vi "GetParameters.vi"(0 "Camera Reference in":refnum<k24>, 1 "error in (no error)":errorcluster) -> (2 "2D ExposureMode (Timed Auto HDR Flash)":enum16{"Timed", "Auto", "HDR", "Flash"}(ring), 3 "2D ExposureTime (0.1-999)":dbl=0.1 min=0.1 max=999.0 step=0.1, 4 "2D Gray Value":i32 min=1 max=999 step=1, 5 "2D Auto-Exposure ROI (x, y, width, height)":T2, 6 "2D Tone Mapping":bool, 7 "2D HDR Exposure Count":i32, 8 "2D HDR Exposure Sequence":T1, 9 "3D Exposure Multiplier":i32, 10 "3D Exposure Sequence":T3, 11 "3D Gain (0-16)":dbl, 12 "Depth Range (lower upper)":cluster{"lower":i32, "upper":i32}, 13 "ROI (x, y, width, height)":T2, 14 "Camera Reference out":refnum<k24>, 15 "error out":errorcluster, 16 "PointCloudSurfaceSmoothing (Off Weak Normal Strong)":u8(ring) items=["Off", "Weak", "Normal", "Strong"], 17 "PointCloudNoiseRemoval (Off Weak Normal Strong)":u8(ring) items=["Off", "Weak", "Normal", "Strong"], 18 "PointCloudOutlierRemoval (Off Weak Normal Strong)":u8(ring) items=["Off", "Weak", "Normal", "Strong"], 19 "Stripe Contrast Threshold (0-100)":i32 min=0 max=100 step=1)   [LabVIEW 2023]
uses:
  C:/Users/mech-mind/Downloads/LabView/MechEyeApiNet.dll
  MechEyeApiNet.dll
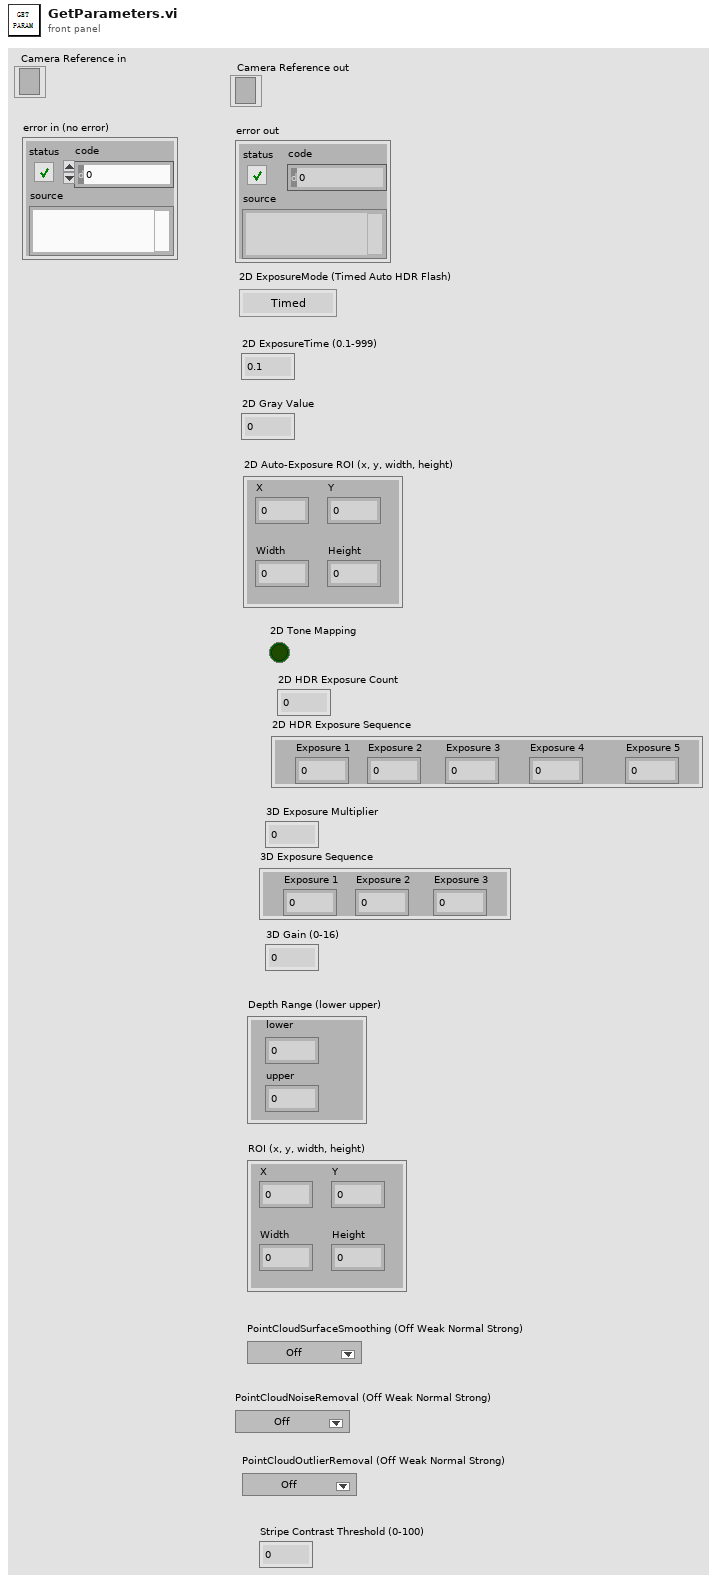
[diagram p1: front panel]
types:
  T1 = cluster{"Exposure 1":dbl, "Exposure 2":dbl, "Exposure 3":dbl, "Exposure 4":dbl, "Exposure 5":dbl}
  T2 = cluster{"X":i32, "Y":i32, "Width":i32, "Height":i32}
  T3 = cluster{"Exposure 1":dbl, "Exposure 2":dbl, "Exposure 3":dbl}
  T4 = cluster{"UpperLeftX":u32, "UpperLeftY":u32, "Width":u64, "Height":u64}
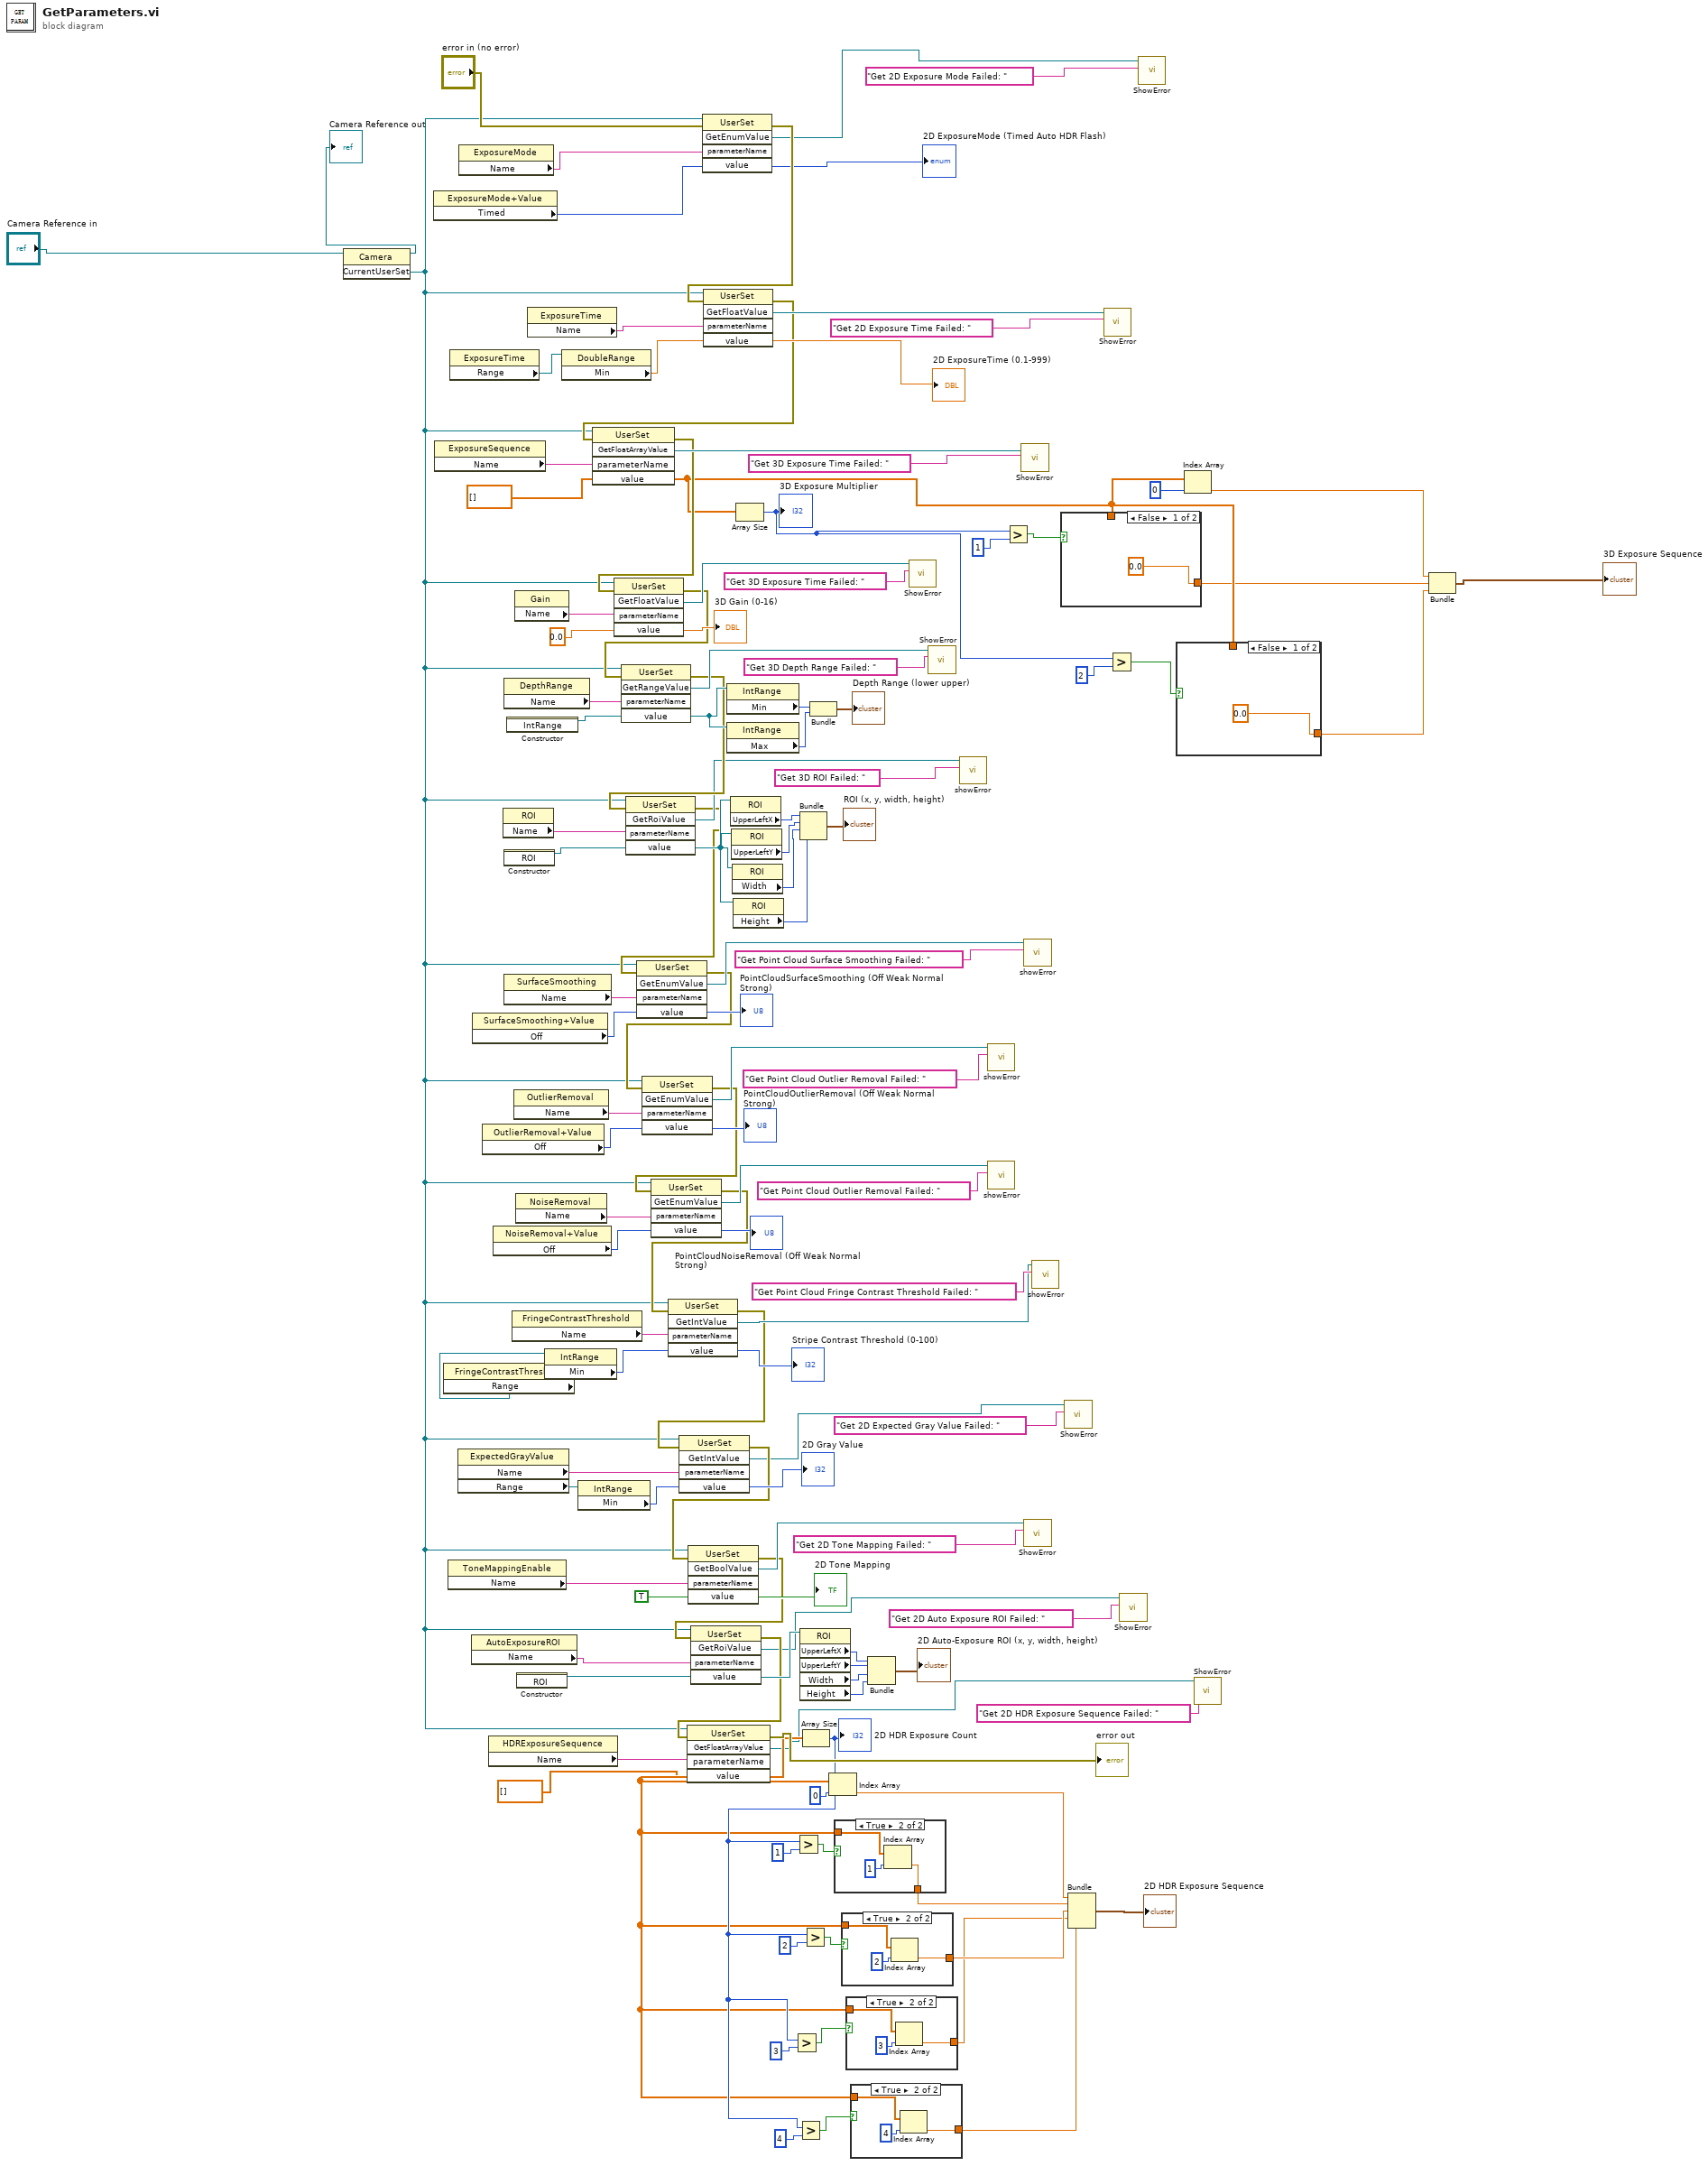
[diagram p0: block diagram]
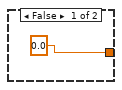
[diagram p2: hidden frame]
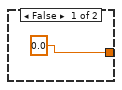
[diagram p3: hidden frame]
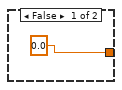
[diagram p4: hidden frame]
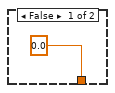
[diagram p5: hidden frame]
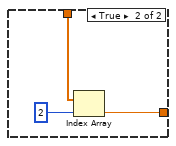
[diagram p6: hidden frame]
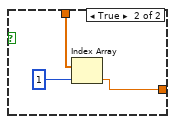
[diagram p7: hidden frame]
diagram:
  n1 = invoke class="Camera" method="CurrentUserSet"(reference="Camera Reference in") -> (reference out=→"Camera Reference out":refnum<k24>, "CurrentUserSet"=w25:refnum<k24>)  [unwired: 2 in, 1 out]
  n2 = property class="ExposureMode+Value"() -> ("Timed"=w120:i32)  [unwired: 2 in, 2 out]
  n3 = property class="ExposureSequence"() -> ("Name"=w117:string)  [unwired: 2 in, 2 out]
  n4 = property class="FringeContrastThreshold"() -> ("Range"=w63:refnum<k24>)  [unwired: 2 in, 2 out]
  n5 = property class="ToneMappingEnable"() -> ("Name"=w42:string)  [unwired: 2 in, 2 out]
  n6 = property class="ExposureTime"() -> ("Range"=w119:refnum<k24>)  [unwired: 2 in, 2 out]
  n7 = property class="ExpectedGrayValue"() -> ("Name"=w46:string, "Range"=w45:refnum<k24>)  [unwired: 2 in, 2 out]
  n8 = property class="ExposureMode"() -> ("Name"=w124:string)  [unwired: 2 in, 2 out]
  n9 = property class="AutoExposureROI"() -> ("Name"=w34:string)  [unwired: 2 in, 2 out]
  n10 = property class="SurfaceSmoothing+Value"() -> ("Off"=w86:i32)  [unwired: 2 in, 2 out]
  n11 = property class="OutlierRemoval+Value"() -> ("Off"=w80:i32)  [unwired: 2 in, 2 out]
  n12 = property class="HDRExposureSequence"() -> ("Name"=w24:string)  [unwired: 2 in, 2 out]
  n13 = property class="NoiseRemoval+Value"() -> ("Off"=w75:i32)  [unwired: 2 in, 2 out]
  n14 = property class="ROI"() -> ("Name"=w97:string)  [unwired: 2 in, 2 out]
  n15 = property class="DepthRange"() -> ("Name"=w108:string)  [unwired: 2 in, 2 out]
  n16 = constructor class="ROI"() -> (reference out=w96:refnum<k24>)  [unwired: 3 in, 2 out]
  n17 = property class="SurfaceSmoothing"() -> ("Name"=w87:string)  [unwired: 2 in, 2 out]
  n18 = constructor class="IntRange"() -> (reference out=w107:refnum<k24>)  [unwired: 3 in, 2 out]
  n19 = property class="FringeContrastThreshold"() -> ("Name"=w64:string)  [unwired: 2 in, 2 out]
  n20 = property class="OutlierRemoval"() -> ("Name"=w81:string)  [unwired: 2 in, 2 out]
  n21 = property class="Gain"() -> ("Name"=w111:string)  [unwired: 2 in, 2 out]
  n22 = property class="NoiseRemoval"() -> ("Name"=w76:string)  [unwired: 2 in, 2 out]
  n23 = constructor class="ROI"() -> (reference out=w27:refnum<k24>)  [unwired: 3 in, 2 out]
  n24 = property class="ExposureTime"() -> ("Name"=w122:string)  [unwired: 2 in, 2 out]
  n25 = property class="IntRange"(reference=w63) -> ("Min"=w62:i32)  [unwired: 1 in, 2 out]
  n26 = property class="DoubleRange"(reference=w119) -> ("Min"=w118:dbl)  [unwired: 1 in, 2 out]
  n27 = property class="IntRange"(reference=w45) -> ("Min"=w44:i32)  [unwired: 1 in, 2 out]
  n28 = invoke class="UserSet" method="GetEnumValue"(reference=w25, error in="error in (no error)", "parameterName"=w124, "value"=w120) -> (error out=w129:errorcluster, "GetEnumValue"=w126:refnum<k24>, "value"=→"2D ExposureMode (Timed Auto HDR Flash)":i32)  [unwired: 1 in, 2 out]
  n29 = invoke class="UserSet" method="GetFloatValue"(reference=w25, error in=w129, "parameterName"=w122, "value"=w118) -> (error out=w100:errorcluster, "GetFloatValue"=w125:refnum<k24>, "value"=→"2D ExposureTime (0.1-999)":dbl)  [unwired: 1 in, 2 out]
  n30 = invoke class="UserSet" method="GetFloatArrayValue"(reference=w25, error in=w100, "parameterName"=w117, "value"=dbl[] [] ("Array")) -> (error out=w99:errorcluster, "GetFloatArrayValue"=w114:refnum<k24>, "value"=w55:dbl[])  [unwired: 1 in, 2 out]
  n31 = invoke class="UserSet" method="GetFloatValue"(reference=w25, error in=w99, "parameterName"=w111, "value"=0.0) -> (error out=w98:errorcluster, "GetFloatValue"=w109:refnum<k24>, "value"=→"3D Gain (0-16)":dbl)  [unwired: 1 in, 2 out]
  n32 = invoke class="UserSet" method="GetRangeValue"(reference=w25, error in=w98, "parameterName"=w108, "value"=w107) -> (error out=w95:errorcluster, "GetRangeValue"=w101:refnum<k24>, "value"=w106:refnum<k24>)  [unwired: 1 in, 2 out]
  n33 = invoke class="UserSet" method="GetRoiValue"(reference=w25, error in=w95, "parameterName"=w97, "value"=w96) -> (error out=w71:errorcluster, "GetRoiValue"=w84:refnum<k24>, "value"=w94:refnum<k24>)  [unwired: 1 in, 2 out]
  n34 = invoke class="UserSet" method="GetEnumValue"(reference=w25, error in=w71, "parameterName"=w87, "value"=w86) -> (error out=w70:errorcluster, "GetEnumValue"=w82:refnum<k24>, "value"=→"PointCloudSurfaceSmoothing (Off Weak Normal Strong)":i32)  [unwired: 1 in, 2 out]
  n35 = invoke class="UserSet" method="GetEnumValue"(reference=w25, error in=w70, "parameterName"=w81, "value"=w80) -> (error out=w69:errorcluster, "GetEnumValue"=w77:refnum<k24>, "value"=→"PointCloudOutlierRemoval (Off Weak Normal Strong)":i32)  [unwired: 1 in, 2 out]
  n36 = invoke class="UserSet" method="GetEnumValue"(reference=w25, error in=w69, "parameterName"=w76, "value"=w75) -> (error out=w67:errorcluster, "GetEnumValue"=w72:refnum<k24>, "value"=→"PointCloudNoiseRemoval (Off Weak Normal Strong)":i32)  [unwired: 1 in, 2 out]
  n37 = invoke class="UserSet" method="GetIntValue"(reference=w25, error in=w67, "parameterName"=w64, "value"=w62) -> (error out=w48:errorcluster, "GetIntValue"=w65:refnum<k24>, "value"=→"Stripe Contrast Threshold (0-100)":i32)  [unwired: 1 in, 2 out]
  n38 = invoke class="UserSet" method="GetIntValue"(reference=w25, error in=w48, "parameterName"=w46, "value"=w44) -> (error out=w40:errorcluster, "GetIntValue"=w38:refnum<k24>, "value"=→"2D Gray Value":i32)  [unwired: 1 in, 2 out]
  n39 = invoke class="UserSet" method="GetBoolValue"(reference=w25, error in=w40, "parameterName"=w42, "value"=TRUE) -> (error out=w35:errorcluster, "GetBoolValue"=w36:refnum<k24>, "value"=→"2D Tone Mapping":bool)  [unwired: 1 in, 2 out]
  n40 = invoke class="UserSet" method="GetRoiValue"(reference=w25, error in=w35, "parameterName"=w34, "value"=w27) -> (error out=w26:errorcluster, "GetRoiValue"=w3:refnum<k24>, "value"=w33:refnum<k24>)  [unwired: 1 in, 2 out]
  n41 = invoke class="UserSet" method="GetFloatArrayValue"(reference=w25, error in=w26, "parameterName"=w24, "value"=dbl[] []) -> (error out=→"error out":errorcluster, "GetFloatArrayValue"=w1:refnum<k24>, "value"=w7:dbl[])  [unwired: 1 in, 2 out]
  n42 = property class="IntRange"(reference=w106) -> ("Min"=w105:i32)  [unwired: 1 in, 2 out]
  n43 = property class="IntRange"(reference=w106) -> ("Max"=w104:i32)  [unwired: 1 in, 2 out]
  n44 = property class="ROI"(reference=w94) -> ("UpperLeftX"=w92:u32)  [unwired: 1 in, 2 out]
  n45 = property class="ROI"(reference=w94) -> ("UpperLeftY"=w91:u32)  [unwired: 1 in, 2 out]
  n46 = property class="ROI"(reference=w94) -> ("Width"=w90:u64)  [unwired: 1 in, 2 out]
  n47 = property class="ROI"(reference=w94) -> ("Height"=w89:u64)  [unwired: 1 in, 2 out]
  n48 = Array Size(array=w55) -> (size(s)=w57:i32)
  "3D Exposure Multiplier" <- w57
  n49 = Bundle("UpperLeftX"=w92, "UpperLeftY"=w91, "Width"=w90, "Height"=w89) -> (→"ROI (x, y, width, height)":T4)  [unwired: 1 in]
  n50 = property class="ROI"(reference=w33) -> ("UpperLeftX"=w31:u32, "UpperLeftY"=w30:u32, "Width"=w29:u64, "Height"=w28:u64)  [unwired: 1 in, 2 out]
  n51 = Array Size(array=w7) -> (size(s)=w8:i32)
  "2D HDR Exposure Count" <- w8
  n52 = Greater?(x=w8, y=3) -> (0:w12:bool)
  n53 = Greater?(x=w8, y=1) -> (0:w20:bool)
  n54 = Greater?(x=w8, y=4) -> (0:w9:bool)
  n55 = Greater?(x=w8, y=2) -> (0:w18:bool)
  n56 = Bundle("Min"=w105, "Max"=w104) -> (→"Depth Range (lower upper)":cluster{"Min":i32, "Max":i32})  [unwired: 1 in]
  n57 = Index Array(array=w7, index=0) -> (element=w16:dbl)
  n58 = case shown="True" w20 {
    tunnel: w7 -> [_ w133]
    tunnel: [0.0 w132] -> w15
    frame False {
    }
    frame True {
      n59 = Index Array(array=w133, index=1) -> (element=w132:dbl)
    }
  }
  n60 = case shown="True" w18 {
    tunnel: w7 -> [_ w137]
    tunnel: [0.0 w136] -> w14
    frame False {
    }
    frame True {
      n61 = Index Array(array=w137, index=2) -> (element=w136:dbl)
    }
  }
  n62 = case shown="True" w12 {
    tunnel: w7 -> [_ w141]
    tunnel: [0.0 w140] -> w11
    frame False {
    }
    frame True {
      n63 = Index Array(array=w141, index=3) -> (element=w140:dbl)
    }
  }
  n64 = case shown="True" w9 {
    tunnel: w7 -> [_ w145]
    tunnel: [0.0 w144] -> w6
    frame False {
    }
    frame True {
      n65 = Index Array(array=w145, index=4) -> (element=w144:dbl)
    }
  }
  n66 = Bundle("UpperLeftX"=w31, "UpperLeftY"=w30, "Width"=w29, "Height"=w28) -> (→"2D Auto-Exposure ROI (x, y, width, height)":T4)  [unwired: 1 in]
  n67 = call "ShowError.vi"("String"="Get 3D Exposure Time Failed: ", "ErrorStatus Refnum in"=w109) -> ()  [unwired: 10 in]
  n68 = call "ShowError.vi"("String"="Get 3D Depth Range Failed: ", "ErrorStatus Refnum in"=w101) -> ()  [unwired: 10 in]
  n69 = call "showError.vi"("String"="Get 3D ROI Failed: ", "ErrorStatus Refnum in"=w84) -> ()  [unwired: 10 in]
  n70 = call "showError.vi"("String"="Get Point Cloud Outlier Removal Failed: ", "ErrorStatus Refnum in"=w77) -> ()  [unwired: 10 in]
  n71 = call "showError.vi"("String"="Get Point Cloud Outlier Removal Failed: ", "ErrorStatus Refnum in"=w72) -> ()  [unwired: 10 in]
  n72 = Greater?(x=w57, y=1) -> (0:w59:bool)
  n73 = call "ShowError.vi"("String"="Get 3D Exposure Time Failed: ", "ErrorStatus Refnum in"=w114) -> ()  [unwired: 10 in]
  n74 = call "showError.vi"("String"="Get Point Cloud Surface Smoothing Failed: ", "ErrorStatus Refnum in"=w82) -> ()  [unwired: 10 in]
  n75 = call "ShowError.vi"("String"="Get 2D Tone Mapping Failed: ", "ErrorStatus Refnum in"=w36) -> ()  [unwired: 10 in]
  n76 = call "showError.vi"("String"="Get Point Cloud Fringe Contrast Threshold Failed: ", "ErrorStatus Refnum in"=w65) -> ()  [unwired: 10 in]
  n77 = case shown="False" w59 {
    tunnel: w55 -> [_ w149]
    tunnel: [0.0 w148] -> w53
    frame False {
    }
    frame True {
      n78 = Index Array(array=w149, index=1) -> (element=w148:dbl)
    }
  }
  n79 = call "ShowError.vi"("String"="Get 2D Expected Gray Value Failed: ", "ErrorStatus Refnum in"=w38) -> ()  [unwired: 10 in]
  n80 = Bundle(w16, w15, w14, w11, w6) -> (→"2D HDR Exposure Sequence":cluster{dbl, dbl, dbl, dbl, dbl})  [unwired: 1 in]
  n81 = call "ShowError.vi"("String"="Get 2D Exposure Time Failed: ", "ErrorStatus Refnum in"=w125) -> ()  [unwired: 10 in]
  n82 = Greater?(x=w57, y=2) -> (0:w56:bool)
  n83 = call "ShowError.vi"("String"="Get 2D Auto Exposure ROI Failed: ", "ErrorStatus Refnum in"=w3) -> ()  [unwired: 10 in]
  n84 = call "ShowError.vi"("String"="Get 2D Exposure Mode Failed: ", "ErrorStatus Refnum in"=w126) -> ()  [unwired: 10 in]
  n85 = case shown="False" w56 {
    tunnel: w55 -> [_ w153]
    tunnel: [0.0 w152] -> w52
    frame False {
    }
    frame True {
      n86 = Index Array(array=w153, index=2) -> (element=w152:dbl)
    }
  }
  n87 = Index Array(array=w55, index=0) -> (element=w54:dbl)
  n88 = call "ShowError.vi"("String"="Get 2D HDR Exposure Sequence Failed: ", "ErrorStatus Refnum in"=w1) -> ()  [unwired: 10 in]
  n89 = Bundle(w54, w53, w52) -> (→"3D Exposure Sequence":cluster{dbl, dbl, dbl})  [unwired: 1 in]
